vi "Set Parameters.vi"(7 "File Level":T1, 8 "error in (no error)":errorcluster, 9 "property values":variant[](array[variant]), 10 "property names":string[](array[string]), 11 "TDMS.lvclass in":refnum<class "TDMS.lvclass">) -> (0 "error out":errorcluster, 3 "TDMS.lvclass out":refnum<class "TDMS.lvclass">)   [LabVIEW 2011, in "TDMS.lvclass"]
uses:
  TDMS.lvclass
  File Level.ctl
  TDMS.lvclass/TDMS.ctl
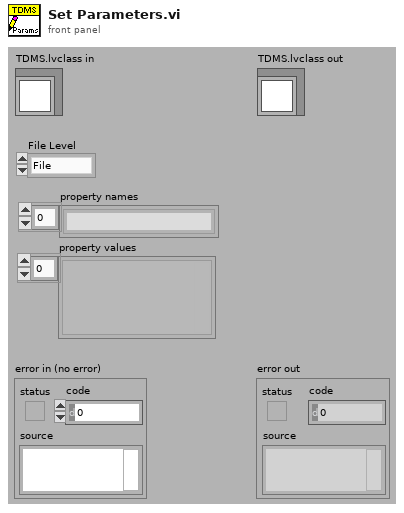
[diagram p1: front panel]
types:
  T1 = typedef "TDMS.lvclass/File Level.ctl" = enum16{"File", "Group", "Channel"}
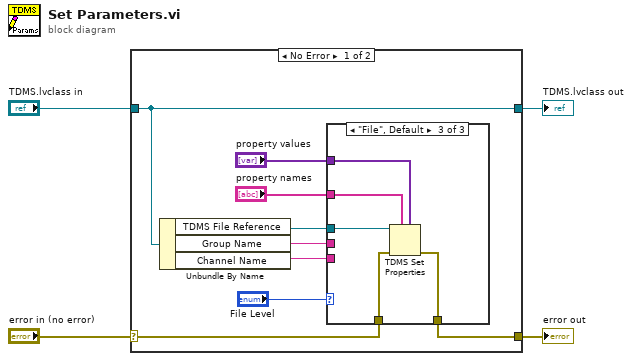
[diagram p0: block diagram]
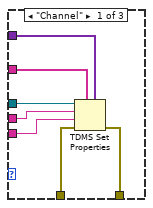
[diagram p2: hidden frame]
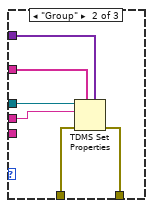
[diagram p3: hidden frame]
diagram:
  n1 = case shown="No Error" "error in (no error)" {
    selector: "error in (no error)" -> [w10 w32]
    tunnel: [w9 w32] -> w3
    tunnel: [w13 w33] -> w1
    tunnel: "TDMS.lvclass in" -> [w13 w33]
    frame No Error {
      n2 = Unbundle By Name(w13) -> ("TDMS File Reference"=w12:refnum<k34>, "Group Name"=w11:string, "Channel Name"=w8:string)
      n3 = case shown="\"File\", Default" "File Level" {
        tunnel: w12 -> [w20 w26 w31]
        tunnel: w11 -> [w19 w25 _]
        tunnel: w10 -> [w17 w24 w30]
        tunnel: [w16 w23 w29] -> w9
        tunnel: w8 -> [w18 _ _]
        tunnel: "property names" -> [w15 w21 w28]
        tunnel: "property values" -> [w14 w22 w27]
        frame "Channel" {
          n4 = TDMS Set Properties(5:w14, 7:w15, 8:w17, 9:w18, 10:w19, 11:w20) -> (0:w16:errorcluster)  [unwired: 3 out]
        }
        frame "Group" {
          n5 = TDMS Set Properties(5:w22, 7:w21, 8:w24, 10:w25, 11:w26) -> (0:w23:errorcluster)  [unwired: 1 in, 3 out]
        }
        frame "File", Default {
          n6 = TDMS Set Properties(5:w27, 7:w28, 8:w30, 11:w31) -> (0:w29:errorcluster)  [unwired: 2 in, 3 out]
        }
      }
    }
    frame Error {
    }
  }
  "error out" <- w3
  "TDMS.lvclass out" <- w1
